vi "Get Network Endpoint Enqueuer.vi"(8 "error in":errorcluster, 11 "MSS Target Actor in":refnum<class "MSS Target Actor.lvclass">) -> (0 "error out":errorcluster, 1 "Connected?":bool, 2 "Enqueuer":refnum<class "Message Enqueuer.lvclass">, 3 "MSS Target Actor out":refnum<class "MSS Target Actor.lvclass">)   [LabVIEW 2024, in "MSS Target Actor.lvlib" / "MSS Target Actor.lvclass"]
uses:
  MSS Target Actor.lvclass
  MSS Target Actor.lvclass/MSS Target Actor.ctl
  <vilib>/ActorFramework/Message Enqueuer/Message Enqueuer.lvclass
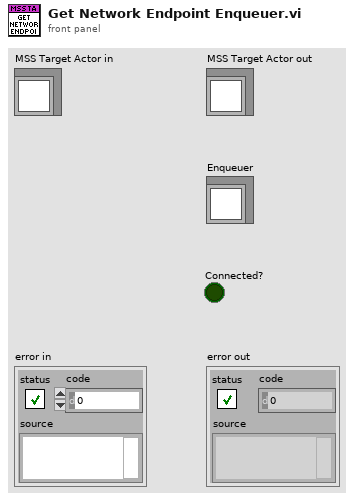
[diagram p1: front panel]
types:
  T1 = map{string, refnum<class "Message Enqueuer.lvclass">}
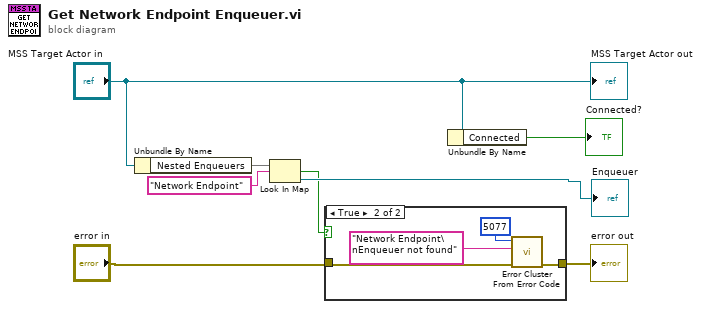
[diagram p0: block diagram]
diagram:
  n1 = Unbundle By Name("MSS Target Actor in") -> ("Nested Enqueuers"=w5:T1)
  n2 = Look In Map(map=w5, key="Network Endpoint") -> (key not found?=w3:bool, value=→"Enqueuer":refnum<class "Message Enqueuer.lvclass">)  [unwired: 1 in]
  n3 = case shown="True" w3 {
    tunnel: "error in" -> [w9 w13]
    tunnel: [w9 w12] -> w7
    frame False {
    }
    frame True {
      n4 = call <vilib>:"Error Cluster From Error Code.vi"("error in (no error)"=w13, "error message (\"\")"="Network Endpoint\nEnqueuer not found" ("error message (\"\")"), "error code (0)"=5077) -> ("error out"=w12:errorcluster)  [unwired: 6 in]
    }
  }
  "error out" <- w7
  n5 = Unbundle By Name("MSS Target Actor in") -> ("Connected"=→"Connected?":bool)
  "MSS Target Actor out" <- "MSS Target Actor in"
